vi "Backgate Array.vi"(11 "Sensors":bool[](array[boolean])) -> (3 "Array":string[](array[string]))   [LabVIEW 2019]
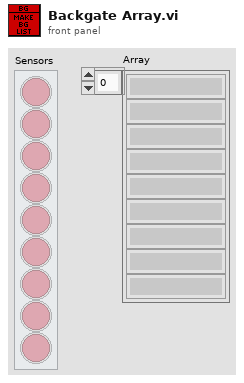
[diagram p1: front panel]
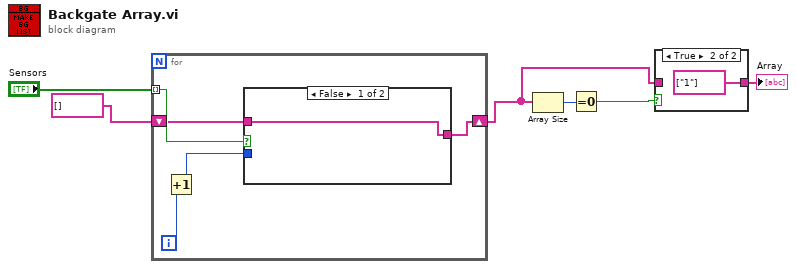
[diagram p0: block diagram]
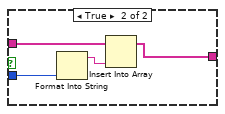
[diagram p3: hidden frame]
diagram:
  n1 = for {
    tunnel: "Sensors" -> [w10] mode=indexing
    shift-right: [w7] -> w1
    shift-left: string[] [] -> [w8]
    i -> [w11]
    n2 = Increment(x=w11) -> (x+1=w9:i32)
    n3 = case shown="False" w10 {
      tunnel: w9 -> [_ w16]
      tunnel: w8 -> [w12 w14]
      tunnel: [w12 w13] -> w7
      frame False {
      }
      frame True {
        n4 = Format Into String(w16) -> (resulting string=w15:string)  [unwired: 3 in, 1 out]
        n5 = Insert Into Array(array=w14, new element=w15) -> (w13:string[])  [unwired: 1 in]
      }
    }
  }
  n6 = Array Size(array=w1) -> (size(s)=w4:i32)
  n7 = Equal To 0?(x=w4) -> (x = 0?=w3:bool)
  n8 = case shown="True" w3 {
    tunnel: [w17 string[] ["1"]] -> w2
    tunnel: w1 -> [w17 _]
    frame False {
    }
    frame True {
    }
  }
  "Array" <- w2
